vi "S4P Data Processing.vi"(0 "S4P File Path":path=path "D:/Luxshare/EBU Project/Testing/Programming/RS ZNB20/ff.s4p") -> (14 "frequency(Hz)":dbl[](array[numeric]), 16 "Sxx_R":dbl[][](array[numeric]), 18 "Sxx_I":dbl[][](array[numeric]), 19 "TXT_Data":string)   [LabVIEW 2011]
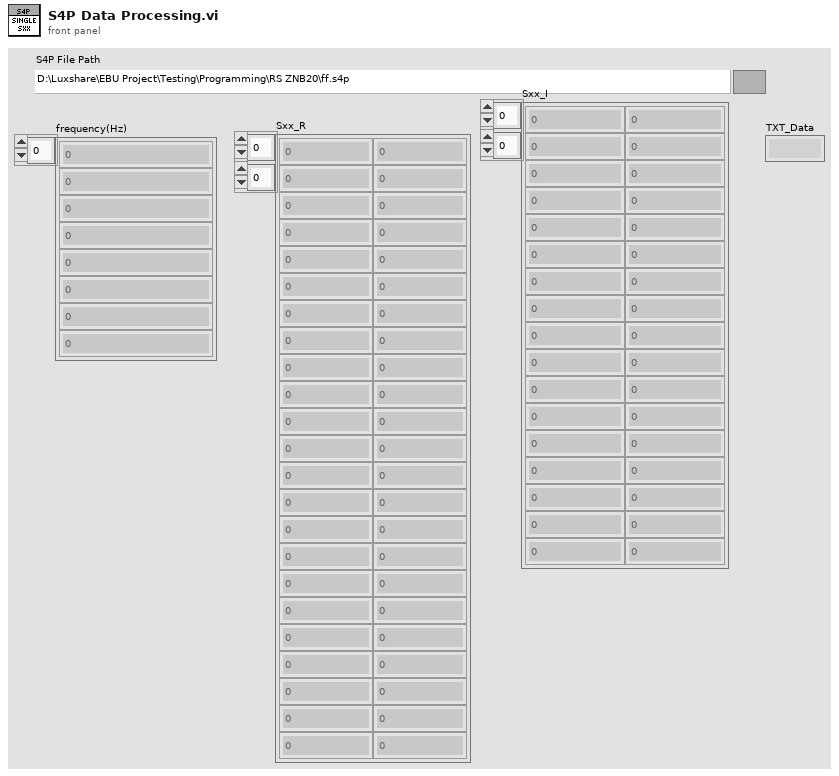
[diagram p1: front panel]
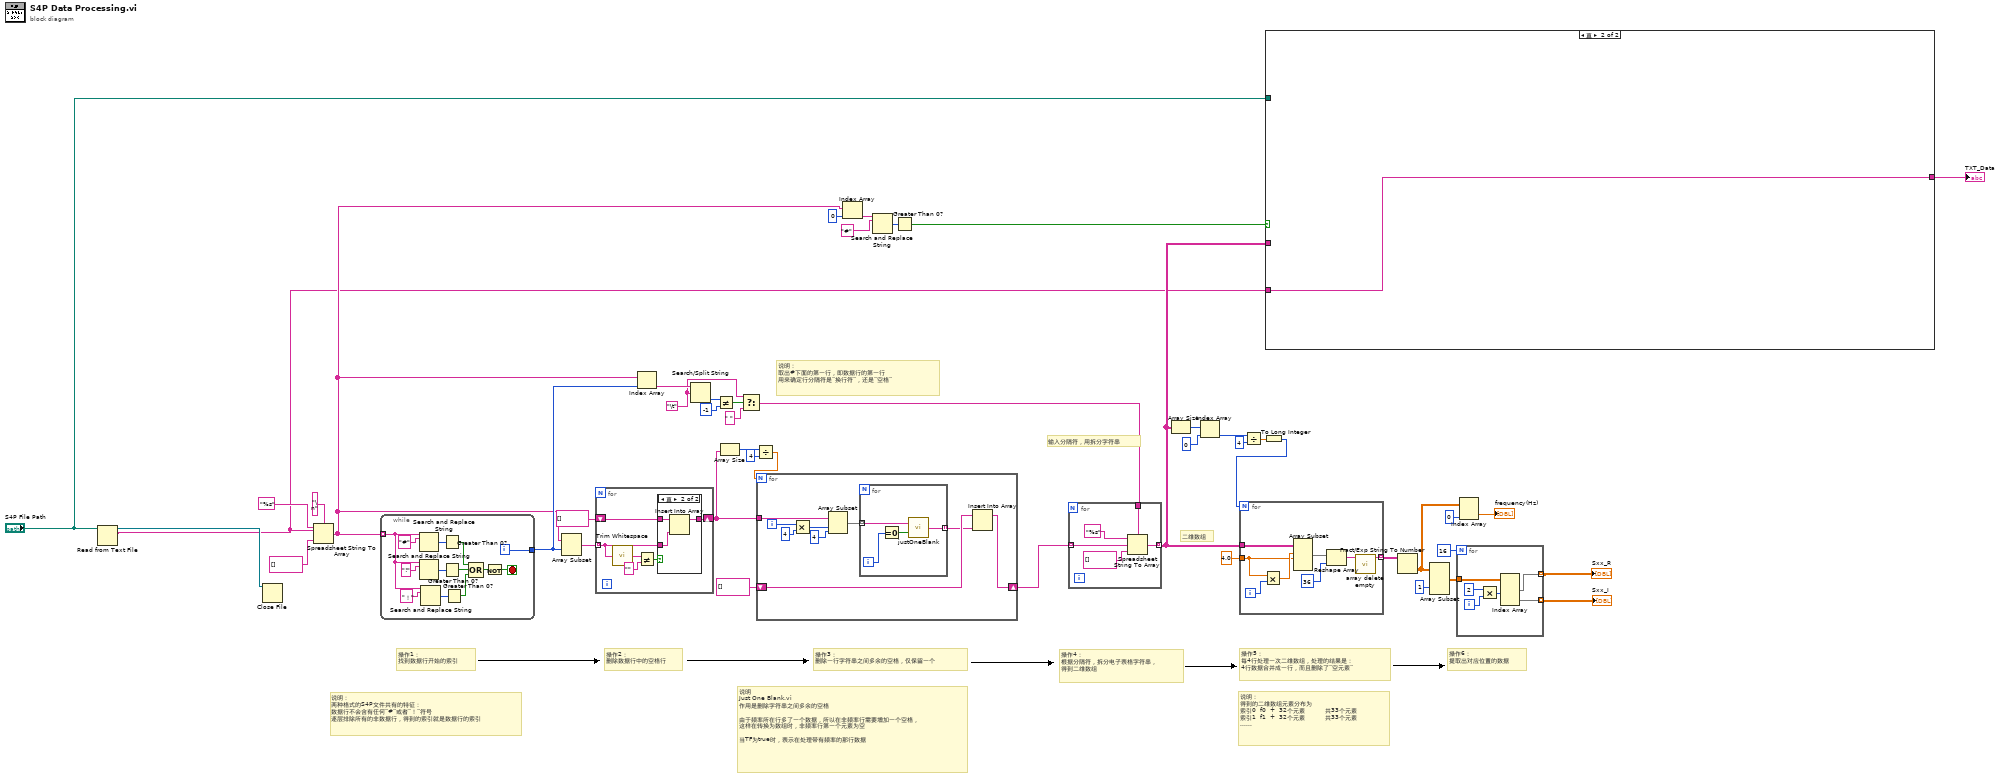
[diagram p0: block diagram]
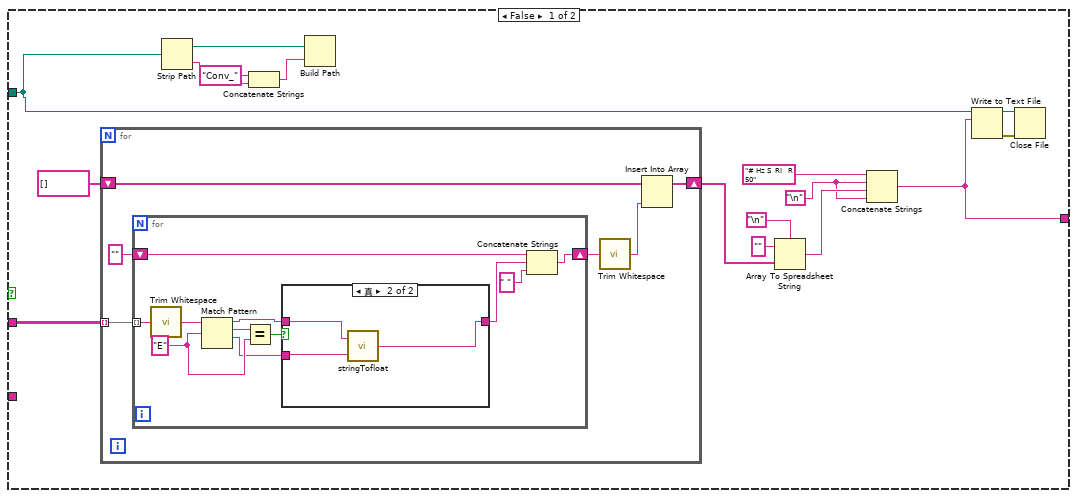
[diagram p2: hidden frame]
diagram:
  w26 = "\t"
  # "说明：\n得到的二维数组元素分布为\n索引0  f0  +  32个元素          共33个元素\n索引1  f1  +  32个元素          共33个元素\n......"
  # "操作6：\n提取出对应位置的数据"
  # "操作5：\n每4行处理一次二维数组，处理的结果是：\n4行数据合并成一行，而且删除了“空元素”"
  # "二维数组"
  # "操作4：\n根据分隔符，拆分电子表格字符串，\n得到二维数组"
  # "操作3：\n删除一行字符串之间多余的空格，仅保留一个"
  # "操作1：\n找到数据行开始的索引"
  # "操作2：\n删除数据行中的空格行"
  # "说明\nJust One Blank.vi\n作用是删除字符串之间多余的空格\n                                                            \n由于频率所在行多了一个数据，所以在非频率行需要增加一个空格，\n这样在转换为数组时，非频率行第一个元素为空\n\n当TF为true时，表示在处理带有频率的那行数据"
  # "输入分隔符，用拆分字符串"
  # "说明：\n两种格式的S4P文件共有的特征：\n数据行不会含有任何“#”或者“！”符号\n逐层排除所有的非数据行，得到的索引就是数据行的索引"
  # "说明：\n取出#下面的第一行，即数据行的第一行\n用来确定行分隔符是“换行符”，还是“空格”"
  n1 = Read from Text File(file (use dialog)="S4P File Path") -> (refnum out=w2:refnum<file>, text=w1:string)  [unwired: 3 in, 2 out]
  n2 = Close File(refnum=w2) -> ()  [unwired: 1 in, 2 out]
  n3 = Spreadsheet String To Array(delimiter (Tab)="\n" ("分隔符(Tab)"), format string="%s" ("格式字符串"), spreadsheet string=w1, array type (2D Dbl)=string[] []) -> (array=w12:string[])
  n4 = while {
    tunnel: w12 -> [w49] mode=indexing
    tunnel: [w47] -> w21
    i -> [w47]
    stop <- w53 stop-if-true
    n5 = Search and Replace String(input string=w49, search string="#" ("搜索字符串")) -> (number of replacements=w58:i32)  [unwired: 6 in, 3 out]
    n6 = Search and Replace String(input string=w49, search string="!" ("搜索字符串")) -> (number of replacements=w57:i32)  [unwired: 6 in, 3 out]
    n7 = Search and Replace String(input string=w49, search string="！" ("搜索字符串")) -> (number of replacements=w50:i32)  [unwired: 6 in, 3 out]
    n8 = Greater Than 0?(x=w58) -> (x > 0?=w55:bool)
    n9 = Greater Than 0?(x=w57) -> (x > 0?=w54:bool)
    n10 = Greater Than 0?(x=w50) -> (x > 0?=w48:bool)
    n11 = Compound Arithmetic op=OR(w55, w54, w48) -> (w52:bool)
    n12 = Not(x=w52) -> (.not. x?=w53:bool)
  }
  n13 = Array Subset(array=w12, index=w21) -> (w16:string[])  [unwired: 1 in]
  n14 = for {
    tunnel: w16 -> [w64] mode=indexing
    shift-right: [w62] -> w14
    shift-left: string[] [] -> [w63]
    n15 = call <vilib>:"Trim Whitespace.vi"("string"=w64) -> ("trimmed string"=w60:string)  [unwired: 1 in]
    n16 = Not Equal?(x=w60, y="") -> (x != y?=w65:bool)
    n17 = case shown="真" w65 {
      tunnel: w64 -> [_ w67]
      tunnel: w63 -> [w66 w69]
      tunnel: [w66 w68] -> w62
      frame False {
      }
      frame True {
        n18 = Insert Into Array(array=w69, new element=w67) -> (w68:string[])  [unwired: 1 in]
      }
    }
  }
  n19 = Index Array(array=w12, index=w21) -> (element=w30:string)
  n20 = Search/Split String(string=w30, search string/char (-)=w26) -> (offset of match=w29:i32)  [unwired: 1 in, 2 out]
  n21 = Not Equal?(x=w29, y=-1) -> (x != y?=w27:bool)
  n22 = Array Size(array=w14) -> (size(s)=w17:i32)
  n23 = Select(t=w26, s=w27, f=" " ("分隔符(Tab)")) -> (s? t:f=w24:string)
  n24 = Divide(x=w17, y=4) -> (x/y=w19:dbl)
  n25 = for {
    N: w19 -> [_]
    tunnel: w14 -> [w78]
    shift-right: [w73] -> w6
    shift-left: string[] [] ("子数组") -> [w74]
    i -> [w77]
    n26 = Multiply(x=w77, y=4) -> (x*y=w75:i32)
    n27 = Array Subset(array=w78, index=w75, length=4 ("长度")) -> (w72:string[])
    n28 = for {
      tunnel: w72 -> [w82] mode=indexing
      tunnel: [w81] -> w71 mode=indexing
      i -> [w80]
      n29 = Equal To 0?(x=w80) -> (x = 0?=w79:bool)
      n30 = call "justOneBlank.vi"("TF"=w79, "input"=w82) -> ("output"=w81:string)
    }
    n31 = Insert Into Array(array=w74, new element=w71) -> (w73:string[])  [unwired: 1 in]
  }
  n32 = Index Array(array=w12, index=0 ("索引")) -> (element=w10:string)
  n33 = Search and Replace String(input string=w10, search string="#" ("搜索字符串")) -> (number of replacements=w8:i32)  [unwired: 6 in, 3 out]
  n34 = Greater Than 0?(x=w8) -> (x > 0?=w7:bool)
  n35 = for {
    tunnel: w6 -> [w87] mode=indexing
    tunnel: [w84] -> w5 mode=indexing
    tunnel: w24 -> [w83]
    n36 = Spreadsheet String To Array(delimiter (Tab)=w83, format string="%s" ("格式字符串"), spreadsheet string=w87, array type (2D Dbl)=string[] []) -> (array=w84:string[])
  }
  n37 = Array Size(array=w5) -> (size(s)=w35:i32[])
  n38 = Index Array(array=w35, index=0 ("索引")) -> (element=w13:i32)
  n39 = Divide(x=w13, y=4) -> (x/y=w32:dbl)
  n40 = To Long Integer(number=w32) -> (32bit integer=w31:i32)
  n41 = for {
    N: w31 -> [_]
    tunnel: w5 -> [w95]
    tunnel: 4.0 ("y") -> [w90]
    tunnel: [w88] -> w41 mode=indexing
    i -> [w94]
    n42 = Multiply(x=w90, y=w94) -> (x*y=w93:dbl)
    n43 = Array Subset(array=w95, index (row)=w93, length (row)=w90) -> (w92:string[][])  [unwired: 2 in]
    n44 = Reshape Array(w92, 36 ("维数大小")) -> (w89:string[])
    n45 = call "array delete empty.vi"("input"=w89) -> ("output"=w88:string[])  [unwired: 10 in]
  }
  n46 = case shown="真" w7 {
    tunnel: w5 -> [w111 _]
    tunnel: "S4P File Path" -> [w96 _]
    tunnel: w1 -> [_ w133]
    tunnel: [w97 w133] -> w4
    frame False {
      w107 = "\n"
      n47 = for {
        tunnel: w111 -> [w117] mode=indexing
        shift-right: [w114] -> w103
        shift-left: string[] [] -> [w115]
        n48 = for {
          tunnel: w117 -> [w128] mode=indexing
          shift-right: [w118] -> w113
          shift-left: "" -> [w121]
          w125 = "E"
          n49 = call <vilib>:"Trim Whitespace.vi"("string"=w128) -> ("trimmed string"=w127:string)  [unwired: 1 in]
          n50 = Match Pattern(string=w127, regular expression=w125) -> (before substring=w123:string, match substring=w126:string, after substring=w122:string)  [unwired: 1 in, 1 out]
          n51 = Equal?(x=w126, y=w125) -> (x = y?=w124:bool)
          n52 = case shown="真" w124 {
            tunnel: w123 -> [w129 w132]
            tunnel: w122 -> [_ w131]
            tunnel: [w129 w130] -> w120
            frame False {
            }
            frame True {
              n53 = call "stringTofloat.vi"("指数"=w131, "系数"=w132) -> ("output"=w130:string)
            }
          }
          n54 = Concatenate Strings(w121, w120, " ") -> (w118:string)
        }
        n55 = call <vilib>:"Trim Whitespace.vi"("string"=w113) -> ("trimmed string"=w112:string)  [unwired: 1 in]
        n56 = Insert Into Array(array=w115, new element=w112) -> (w114:string[])  [unwired: 1 in]
      }
      n57 = Strip Path(path=w96) -> (stripped path=w101:path, name=w100:string)
      n58 = Concatenate Strings("Conv_" ("字符串"), w100) -> (w98:string)
      n59 = Build Path(base path=w101, name or relative path=w98) -> ()  [unwired: 1 out]
      n60 = Array To Spreadsheet String(delimiter (Tab)="\n", array=w103, 3:"" ("格式字符串")) -> (spreadsheet string=w108:string)
      n61 = Concatenate Strings("# Hz S  RI   R 50", w107, w108, w107) -> (w97:string)
      n62 = Write to Text File(file (use dialog)=w96, text=w97) -> (refnum out=w106:refnum<file>, error out=w105:errorcluster)  [unwired: 2 in, 1 out]
      n63 = Close File(refnum=w106, error in=w105) -> ()  [unwired: 2 out]
    }
    frame True {
    }
  }
  "TXT_Data" <- w4
  n64 = Fract/Exp String To Number(string=w41) -> (number=w40:dbl[][])  [unwired: 3 in, 1 out]
  n65 = Array Subset(array=w40, index (col)=1 ("索引")) -> (w38:dbl[][])  [unwired: 3 in]
  n66 = for {
    N: 16 -> [_]
    tunnel: w38 -> [w139]
    tunnel: [w135] -> w23 mode=indexing
    tunnel: [w134] -> w22 mode=indexing
    i -> [w138]
    n67 = Multiply(x=2, y=w138) -> (x*y=w136:i32)
    n68 = Index Array(array=w139, index (col) #1=w136) -> (element #1=w135:dbl[], element #2=w134:dbl[])  [unwired: 3 in]
  }
  "Sxx_R" <- w23
  "Sxx_I" <- w22
  n69 = Index Array(array=w40, index (col)=0 ("禁用的索引 (列)")) -> (element=→"frequency(Hz)":dbl[])  [unwired: 1 in]
